vi "Ascii to Hex (2Byte) (조향각만 _ 문자열 반전추가).vi"(2 "Ascii 1":string) -> (0 "Ascii 2":string, 1 "Decimal":i16)   [LabVIEW 2016]
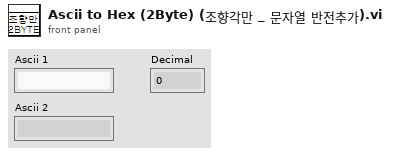
[diagram p1: front panel]
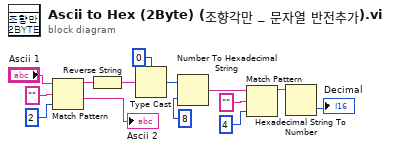
[diagram p0: block diagram]
diagram:
  n1 = Match Pattern(string="Ascii 1", regular expression="" ("정규식"), offset (0)=2 ("길이(나머지)")) -> (before substring=w1:string, after substring=→"Ascii 2":string)  [unwired: 2 out]
  n2 = Reverse String(1:w1) -> (0:w2:string)
  n3 = Type Cast(type=0 ("길이(나머지)"), x=w2) -> (*(type *) &x=w14:i32)
  n4 = Number To Hexadecimal String(1:i16 8 ("폭(-)"), 2:w14) -> (0:w9:string)
  n5 = Match Pattern(string=w9, regular expression="" ("정규식"), offset (0)=4 ("길이(나머지)")) -> (before substring=w4:string)  [unwired: 3 out]
  n6 = Hexadecimal String To Number(string=w4) -> (number=→"Decimal":u32)  [unwired: 2 in, 1 out]
